vi "SUPPORT_ButtonColorPicker.vi"() -> ()   [LabVIEW 2019, in "Menu Button.xctl"]
doc: "JSMA Module Template - Top Level UI 0.2.0.4\nRob Humfeld - Jet Engineering\nCopyright (c) 2019, Jet Engineering"
uses:
  Menu Button.xctl
panel:
  in  "Color 4":string[](array[string])=["500050", "500050"]
  in  "Color 7":string[](array[string])=["000C2B", "000C2B"]
  in  "Color 6":string[](array[string])=["000C2B", "000C2B"]
  in  "Color 5":string[](array[string])=["000C2B", "000C2B"]
  in  "Color 7":bool caption="Button 1"
  in  "Color 6":bool caption="Button 1"
  in  "Color 5":bool caption="Button 1"
  in  "Color 4":bool caption="Button 1"
  out "Color 0":string[](array[string])=["00195B", "00195B"]
  out "Color 3":string[](array[string])=["3E000B", "3E000B"]
  out "Color 2":string[](array[string])=["730013", "730013"]
  out "Color 1":string[](array[string])=["000C2B", "000C2B"]
  in  "Color 3":bool caption="Button 1"
  in  "Color 2":bool caption="Button 1"
  in  "Color 1":bool caption="Button 1"
  in  "Color 0":bool caption="Button 1"
  out "Array":string[](array[string])=["195B", "195B", "5B1C", "5B1C", "C2D", "C2D", "2D0E", "2D0E"]
  in  "System Setup":bool caption="Button 1"
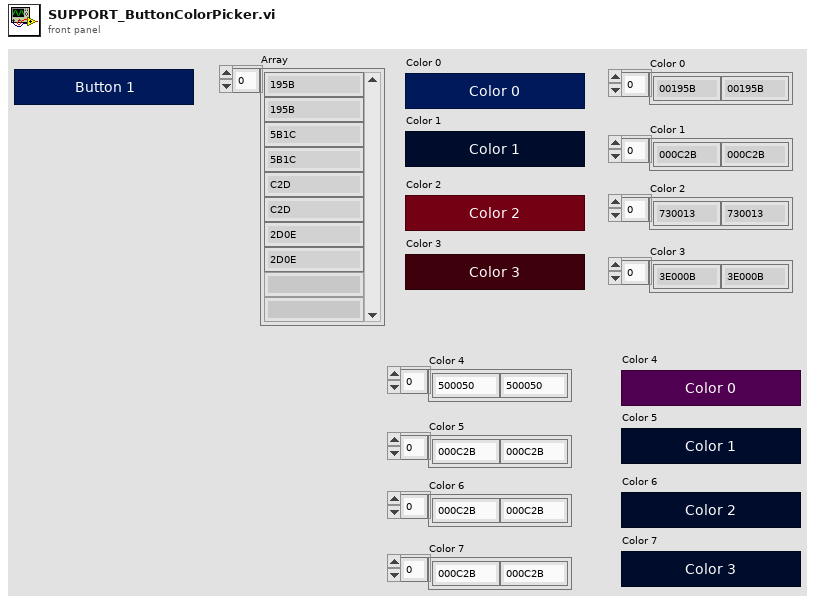
[diagram p1: front panel]
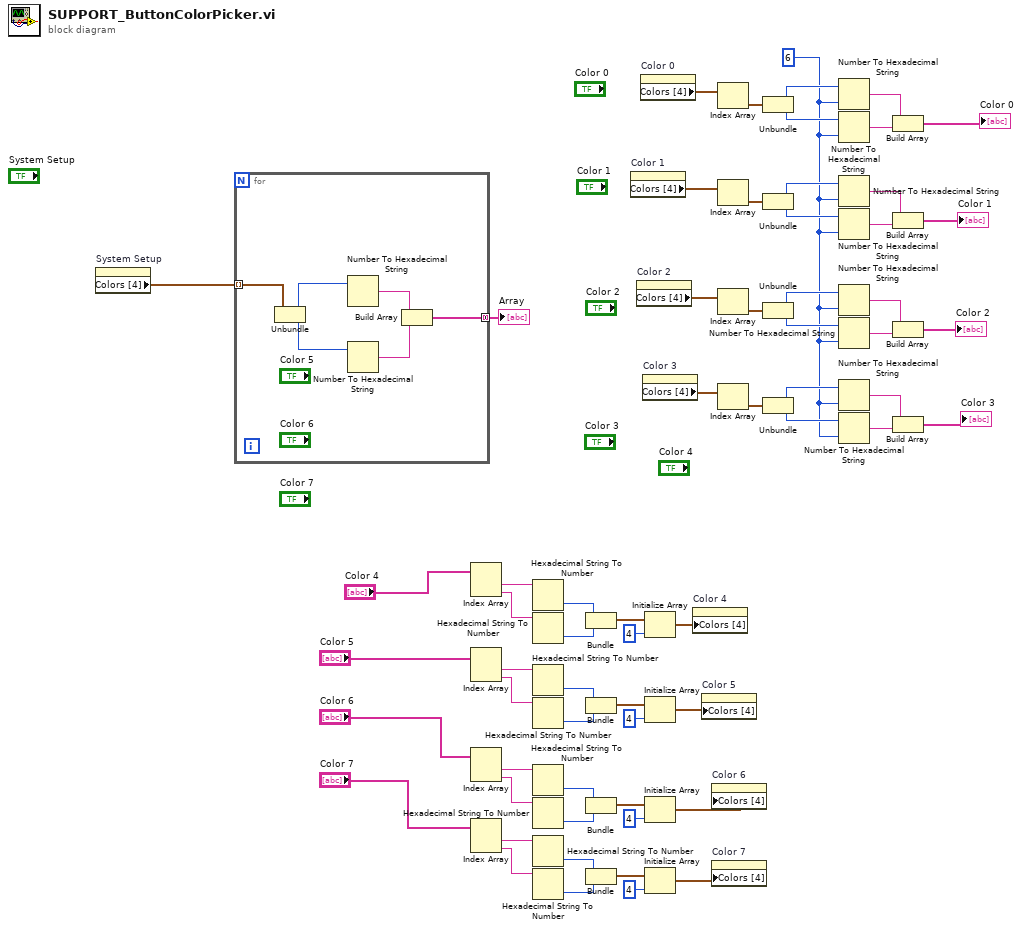
[diagram p0: block diagram]
diagram:
  w33 = i16 6 ("width (-)")
  n1 = property on="System Setup" class="Bool (strict)"() -> ("Colors [4]"=w63:cluster{u32, u32}[])  [unwired: 2 in, 2 out]
  n2 = for {
    tunnel: w63 -> [w69] mode=indexing
    tunnel: [w64] -> w62 mode=concatenating
    n3 = Unbundle(w69) -> (w68:u32, w67:u32)
    n4 = Number To Hexadecimal String(2:w68) -> (0:w66:string)  [unwired: 1 in]
    n5 = Number To Hexadecimal String(2:w67) -> (0:w65:string)  [unwired: 1 in]
    n6 = Build Array(w66, w65) -> (w64:string[])
  }
  "Array" <- w62
  n7 = Index Array(array="Color 4") -> (element #1=w25:string, element #2=w31:string)  [unwired: 2 in]
  n8 = Index Array(array="Color 5") -> (element #1=w24:string, element #2=w19:string)  [unwired: 2 in]
  n9 = Index Array(array="Color 6") -> (element #1=w13:string, element #2=w18:string)  [unwired: 2 in]
  n10 = Index Array(array="Color 7") -> (element #1=w12:string, element #2=w7:string)  [unwired: 2 in]
  n11 = Hexadecimal String To Number(string=w25) -> (number=w29:u32)  [unwired: 2 in, 1 out]
  n12 = Hexadecimal String To Number(string=w31) -> (number=w30:u32)  [unwired: 2 in, 1 out]
  n13 = Hexadecimal String To Number(string=w24) -> (number=w21:u32)  [unwired: 2 in, 1 out]
  n14 = Hexadecimal String To Number(string=w19) -> (number=w20:u32)  [unwired: 2 in, 1 out]
  n15 = Hexadecimal String To Number(string=w13) -> (number=w16:u32)  [unwired: 2 in, 1 out]
  n16 = Hexadecimal String To Number(string=w18) -> (number=w17:u32)  [unwired: 2 in, 1 out]
  n17 = Hexadecimal String To Number(string=w12) -> (number=w9:u32)  [unwired: 2 in, 1 out]
  n18 = Hexadecimal String To Number(string=w7) -> (number=w8:u32)  [unwired: 2 in, 1 out]
  n19 = Bundle(w29, w30) -> (w28:cluster{u32, u32})  [unwired: 1 in]
  n20 = Bundle(w21, w20) -> (w22:cluster{u32, u32})  [unwired: 1 in]
  n21 = Bundle(w16, w17) -> (w15:cluster{u32, u32})  [unwired: 1 in]
  n22 = Bundle(w9, w8) -> (w10:cluster{u32, u32})  [unwired: 1 in]
  n23 = property on="Color 1" class="Bool (strict)"() -> ("Colors [4]"=w61:cluster{u32, u32}[])  [unwired: 2 in, 2 out]
  n24 = property on="Color 2" class="Bool (strict)"() -> ("Colors [4]"=w50:cluster{u32, u32}[])  [unwired: 2 in, 2 out]
  n25 = property on="Color 0" class="Bool (strict)"() -> ("Colors [4]"=w37:cluster{u32, u32}[])  [unwired: 2 in, 2 out]
  n26 = property on="Color 3" class="Bool (strict)"() -> ("Colors [4]"=w38:cluster{u32, u32}[])  [unwired: 2 in, 2 out]
  n27 = Initialize Array(w28, 4 ("dimension size")) -> (w26:cluster{u32, u32}[])
  n28 = Initialize Array(w22, 4 ("dimension size")) -> (w1:cluster{u32, u32}[])
  n29 = Initialize Array(w15, 4 ("dimension size")) -> (w3:cluster{u32, u32}[])
  n30 = Initialize Array(w10, 4 ("dimension size")) -> (w2:cluster{u32, u32}[])
  n31 = property on="Color 4" class="Bool (strict)"("Colors [4]"=w26) -> ()  [unwired: 2 in, 2 out]
  n32 = property on="Color 5" class="Bool (strict)"("Colors [4]"=w1) -> ()  [unwired: 2 in, 2 out]
  n33 = property on="Color 6" class="Bool (strict)"("Colors [4]"=w3) -> ()  [unwired: 2 in, 2 out]
  n34 = property on="Color 7" class="Bool (strict)"("Colors [4]"=w2) -> ()  [unwired: 2 in, 2 out]
  n35 = Index Array(array=w37) -> (element=w43:cluster{u32, u32})  [unwired: 1 in]
  n36 = Index Array(array=w61) -> (element=w55:cluster{u32, u32})  [unwired: 1 in]
  n37 = Index Array(array=w50) -> (element=w54:cluster{u32, u32})  [unwired: 1 in]
  n38 = Index Array(array=w38) -> (element=w44:cluster{u32, u32})  [unwired: 1 in]
  n39 = Unbundle(w43) -> (w39:u32, w40:u32)
  n40 = Unbundle(w55) -> (w60:u32, w59:u32)
  n41 = Unbundle(w54) -> (w34:u32, w51:u32)
  n42 = Unbundle(w44) -> (w48:u32, w47:u32)
  n43 = Number To Hexadecimal String(1:w33, 2:w39) -> (0:w41:string)
  n44 = Number To Hexadecimal String(1:w33, 2:w40) -> (0:w42:string)
  n45 = Number To Hexadecimal String(1:w33, 2:w60) -> (0:w58:string)
  n46 = Number To Hexadecimal String(1:w33, 2:w59) -> (0:w57:string)
  n47 = Number To Hexadecimal String(1:w33, 2:w34) -> (0:w52:string)
  n48 = Number To Hexadecimal String(1:w33, 2:w51) -> (0:w53:string)
  n49 = Number To Hexadecimal String(1:w33, 2:w48) -> (0:w46:string)
  n50 = Number To Hexadecimal String(1:w33, 2:w47) -> (0:w45:string)
  n51 = Build Array(w41, w42) -> (→"Color 0":string[])
  n52 = Build Array(w58, w57) -> (→"Color 1":string[])
  n53 = Build Array(w52, w53) -> (→"Color 2":string[])
  n54 = Build Array(w46, w45) -> (→"Color 3":string[])
